vi "Discover Tests.vi"(8 "error in (no error)":errorcluster, 11 "Test Runner in":refnum<class "Test Runner.lvclass">) -> (0 "error out":errorcluster, 3 "Test Runner out":refnum<class "Test Runner.lvclass">)   [LabVIEW 2013, in "Caraya.lvlib" / "Test Runner.lvclass"]
uses:
  Test Runner.lvclass
  Test Runner.lvclass/Test Runner.ctl
  Test/Test.lvclass
  Caraya.lvlib
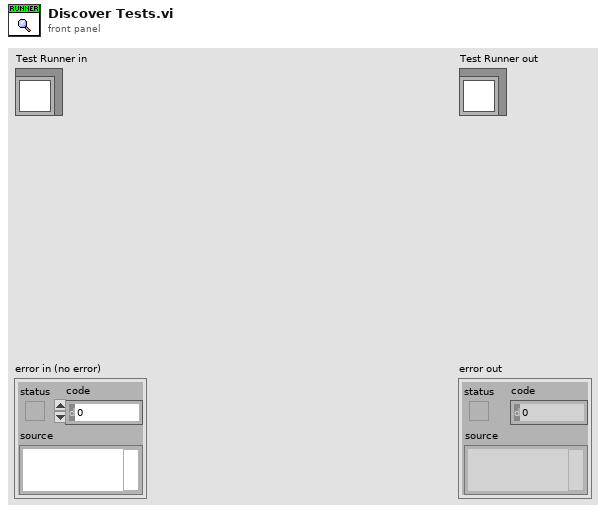
[diagram p1: front panel]
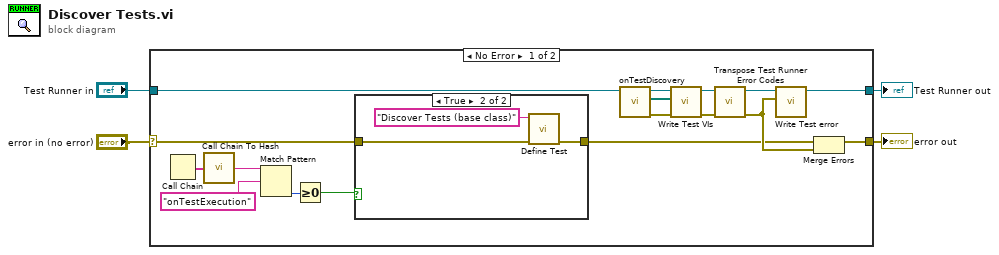
[diagram p0: block diagram]
diagram:
  n1 = case shown="No Error" "error in (no error)" {
    selector: "error in (no error)" -> [w11 w27]
    tunnel: [w20 w27] -> w4
    tunnel: "Test Runner in" -> [w21 w26]
    tunnel: [w19 w26] -> w2
    frame No Error {
      n2 = Call Chain() -> (call chain=w9:string[])
      n3 = call "Call Chain To Hash.vi"("VI Call Chain"=w9) -> ("Key"=w8:string)
      n4 = Match Pattern(string=w8, regular expression="onTestExecution") -> (offset past match=w6:i32)  [unwired: 1 in, 3 out]
      n5 = Greater Or Equal To 0?(x=w6) -> (x >= 0?=w5:bool)
      n6 = case shown="True" w5 {
        tunnel: w11 -> [w22 w25]
        tunnel: [w22 w24] -> w10
        frame False {
        }
        frame True {
          n7 = call "Define Test.vi"("error in (no error)"=w25, "Label (VI Title)"="Discover Tests (base class)") -> ("error out"=w24:errorcluster)  [unwired: 9 in]
        }
      }
      n8 = call-dynamic "onTestDiscovery.vi"("Test Runner in"=w21) -> ("error out"=w13:errorcluster, "Tests VIs"=w14:path[], "Test Runner out"=w15:refnum<class "Test Runner.lvclass">)  [unwired: 8 in]
      n9 = call "Write Test VIs.vi"("error in (no error)"=w13, "Test VIs"=w14, "Test Runner in"=w15) -> ("error out"=w12:errorcluster, "Test Runner out"=w18:refnum<class "Test Runner.lvclass">)  [unwired: 7 in]
      n10 = call-dynamic "Transpose Test Runner Error Codes.vi"("error in (no error)"=w12, "Test Runner in"=w18) -> ("error out"=w16:errorcluster, "Test Runner out"=w17:refnum<class "Test Runner.lvclass">)  [unwired: 8 in]
      n11 = call "Write Test error.vi"("Test error"=w16, "Test Runner in"=w17) -> ("Test Runner out"=w19:refnum<class "Test Runner.lvclass">)  [unwired: 9 in]
      n12 = Merge Errors(w10, w16) -> (w20:errorcluster)
    }
    frame Error {
    }
  }
  "error out" <- w4
  "Test Runner out" <- w2
